vi "Excel Get Data Specified Field.vi"(4 "error in (no error)":errorcluster, 5 "SheetName":string="Sheet1", 7 "Start and End":T1={"Start Row"=1, "Start Column"=1, "End Row"=1, "End Column"=51}) -> (0 "error out":errorcluster, 2 "data":string[][](array[string])=[["0", "0", "0", "0", "0", "0", "0", "0", "0", "0", "0", "0", "0", "0", "0", "0", "0", "0", "0", "0", "0", "0", "0", "0", "0", "0", "0", "0", "0"]], 3 "array":dbl[][](array[numeric]))   [LabVIEW 2014]
panel:
  out "error out 2":errorcluster
  in  "Excel._Worksheet 2":refnum<k7>
  in  "Array":string[][](array[string])
  in  "Excel._Worksheet":refnum<k7>
  in  "Excel._Application":refnum<k7>
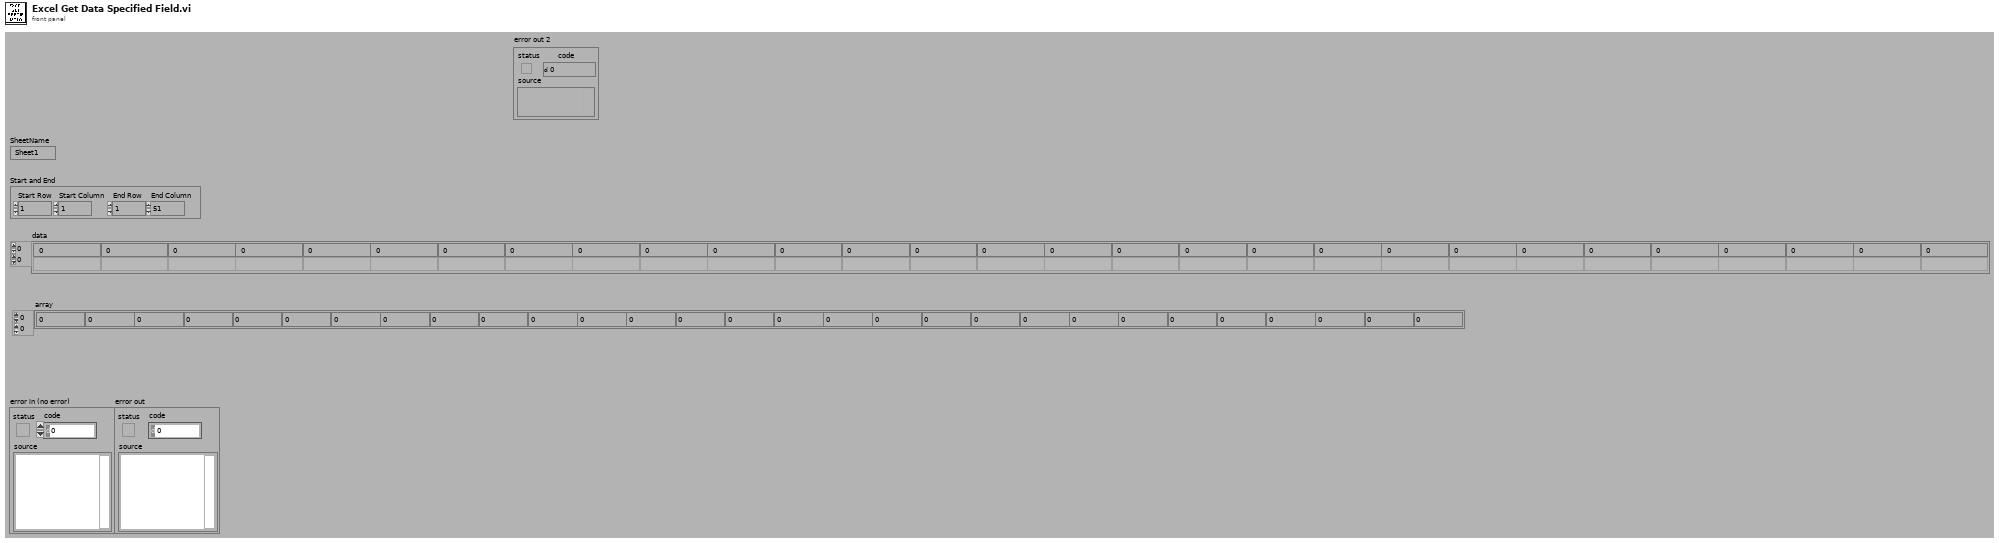
[diagram p1: front panel]
types:
  T1 = cluster{"Start Row":i32, "Start Column":i32, "End Row":i32, "End Column":i32}
  T2 = enum16{"open", "open or create", "create or replace", "create", "open (read only)"}
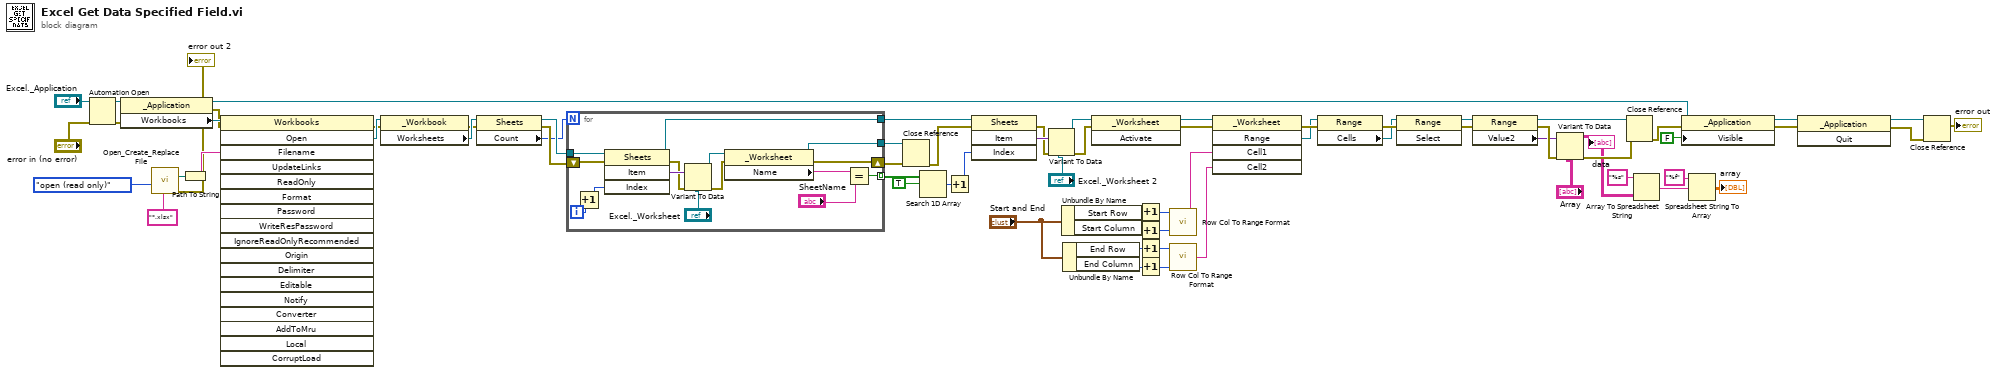
[diagram p0: block diagram]
diagram:
  n1 = Automation Open(error in (no error)="error in (no error)", Automation Refnum="Excel._Application") -> (Automation Refnum=w66:refnum<k7>, error out=w65:errorcluster)  [unwired: 2 in]
  n2 = property class="_Application"(reference=w66, error in=w65) -> (reference out=w56:refnum<k7>, error out=w59:errorcluster, "Workbooks"=w60:refnum<k7>)
  n3 = call <vilib>:"Open_Create_Replace File.vi"("pattern"="*.xlsx", "function (open:0)"=T2."open (read only)") -> ("error out"=→"error out 2":errorcluster, "new file path"=w28:path)  [unwired: 6 in, 2 out]
  n4 = Path To String(path=w28) -> (string=w9:string)
  n5 = invoke class="Workbooks" method="Open"(reference=w60, error in=w59, "Filename"=w9) -> (error out=w57:errorcluster, "Open"=w58:refnum<k7>)  [unwired: 15 in, 16 out]
  n6 = property class="_Workbook"(reference=w58, error in=w57) -> (error out=w47:errorcluster, "Worksheets"=w48:refnum<k7>)  [unwired: 1 out]
  n7 = property class="Sheets"(reference=w48, error in=w47) -> (reference out=w46:refnum<k7>, error out=w43:errorcluster, "Count"=w6:i32)
  n8 = for {
    N: w6 -> [_]
    tunnel: w46 -> [w83]
    shift-right: [w74] -> w39
    shift-left: w43 -> [w82]
    tunnel: [w75] -> w40 mode=indexing
    tunnel: [w73] -> w41
    tunnel: [w72] -> w37
    i -> [w70]
    n9 = Increment(x=w70) -> (x+1=w69:i32)
    n10 = invoke class="Sheets" method="Item"(reference=w83, error in=w82, "Index"=w69) -> (reference out=w73:refnum<k7>, error out=w79:errorcluster, "Item"=w81:variant)  [unwired: 1 in, 1 out]
    n11 = Variant To Data(error in=w79, type="Excel._Worksheet", Variant=w81) -> (data=w77:refnum<k7>, error out=w78:errorcluster)
    n12 = property class="_Worksheet"(reference=w77, error in=w78) -> (reference out=w72:refnum<k7>, error out=w74:errorcluster, "Name"=w76:string)
    n13 = Equal?(x=w76, y="SheetName") -> (x = y?=w75:bool)
  }
  n14 = Close Reference(reference=w37, error in (no error)=w39) -> (error out=w38:errorcluster)
  n15 = Search 1D Array(1D array=w40, element=TRUE) -> (index of element=w44:i32)  [unwired: 1 in]
  n16 = Increment(x=w44) -> (x+1=w7:i32)
  n17 = invoke class="Sheets" method="Item"(reference=w41, error in=w38, "Index"=w7) -> (error out=w63:errorcluster, "Item"=w64:variant)  [unwired: 1 in, 2 out]
  n18 = Variant To Data(error in=w63, type="Excel._Worksheet 2", Variant=w64) -> (data=w36:refnum<k7>, error out=w62:errorcluster)
  n19 = Unbundle By Name("Start and End") -> ("Start Row"=w21:i32, "Start Column"=w20:i32)
  n20 = Unbundle By Name("Start and End") -> ("End Row"=w19:i32, "End Column"=w18:i32)
  n21 = invoke class="_Worksheet" method="Activate"(reference=w36, error in=w62) -> (reference out=w26:refnum<k7>, error out=w25:errorcluster)  [unwired: 1 in, 1 out]
  n22 = Increment(x=w21) -> (x+1=w23:i32)
  n23 = Increment(x=w20) -> (x+1=w24:i32)
  n24 = Increment(x=w19) -> (x+1=w17:i32)
  n25 = Increment(x=w18) -> (x+1=w16:i32)
  n26 = call "Row Col To Range Format.vi"("Column"=w24, "Row"=w23) -> ("Output String"=w15:string)
  n27 = call "Row Col To Range Format.vi"("Column"=w16, "Row"=w17) -> ("Output String"=w14:string)
  n28 = invoke class="_Worksheet" method="Range"(reference=w26, error in=w25, "Cell1"=w15, "Cell2"=w14) -> (error out=w13:errorcluster, "Range"=w12:refnum<k7>)  [unwired: 1 in, 3 out]
  n29 = property class="Range"(reference=w12, error in=w13) -> (error out=w55:errorcluster, "Cells"=w35:refnum<k7>)  [unwired: 1 out]
  n30 = invoke class="Range" method="Select"(reference=w35, error in=w55) -> (reference out=w54:refnum<k7>, error out=w53:errorcluster)  [unwired: 1 in, 1 out]
  n31 = property class="Range"(reference=w54, error in=w53) -> (reference out=w51:refnum<k7>, error out=w52:errorcluster, "Value2"=w8:variant)
  n32 = Variant To Data(error in=w52, type="Array", Variant=w8) -> (data=w11:string[][], error out=w50:errorcluster)
  "data" <- w11
  n33 = Close Reference(reference=w51, error in (no error)=w50) -> (error out=w49:errorcluster)
  n34 = Array To Spreadsheet String(array=w11, 3:"%s" ("format string")) -> (spreadsheet string=w32:string)  [unwired: 1 in]
  n35 = property class="_Application"(reference=w56, error in=w49, "Visible"=FALSE) -> (reference out=w5:refnum<k7>, error out=w4:errorcluster)
  n36 = Spreadsheet String To Array(format string="%f", spreadsheet string=w32) -> (array=→"array":dbl[][])  [unwired: 2 in]
  n37 = invoke class="_Application" method="Quit"(reference=w5, error in=w4) -> (reference out=w3:refnum<k7>, error out=w2:errorcluster)  [unwired: 1 in, 1 out]
  n38 = Close Reference(reference=w3, error in (no error)=w2) -> (error out=→"error out":errorcluster)
